vi "Clear Test Executive.vi"(8 "error in (no error)":errorcluster, 11 "Test Executive Builder Model in":refnum<class "Test Executive Builder Model.lvclass">) -> (0 "error out":errorcluster, 3 "Test Executive Builder Model out":refnum<class "Test Executive Builder Model.lvclass">, 5 "Unique ID":string)   [LabVIEW 2017, in "Test Executive Builder Model.lvclass"]
uses:
  <vilib>/gpm_packages/@cs/Test-executive-builder/Source/Test Executive Builder Model/Test Executive Builder Model/Test Executive Builder Model.lvclass
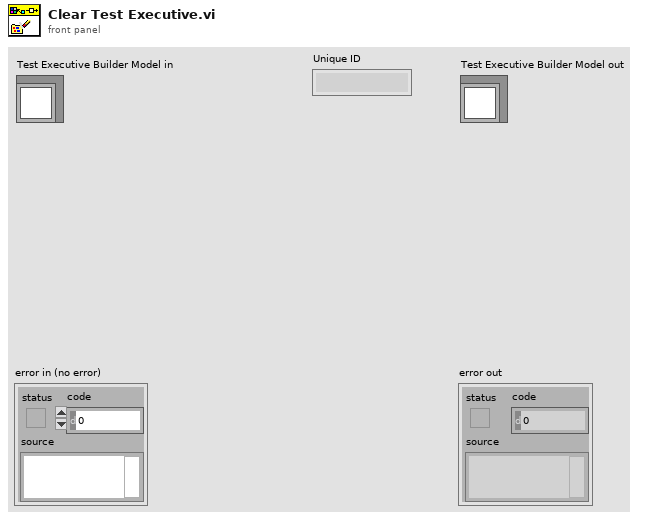
[diagram p1: front panel]
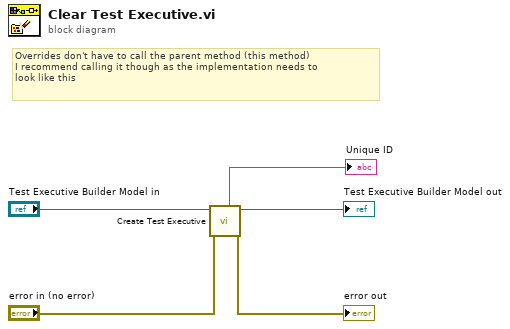
[diagram p0: block diagram]
diagram:
  # "Overrides don't have to call the parent method (this method)\nI recommend calling it though as the implementation needs to\nlook like this"
  n1 = call-dynamic "Create Test Executive.vi"("error in (no error)"="error in (no error)", "Test Executive Builder Model in"="Test Executive Builder Model in") -> ("error out"=→"error out":errorcluster, "Test Executive Builder Model out"=→"Test Executive Builder Model out":refnum<class "Test Executive Builder Model.lvclass">, "Unique ID"=→"Unique ID":string)  [unwired: 7 in]
